vi "Scan_ctrl.vi"(0 "Scan Set up":T4={"Scan Type"=0, "Collection Information File Path"=path "", "Chemical"="Water", "Comments"="", "Collection Time / s"=60, "Number Acquires"=3, "How long to acquire"=75000000} {"Scan Type" items=["Normal Collection - 1 Colour", "Normal Collection - 2 Colour", "Delay Scan - 2 colour", "Accurate Delay Scan - 2 Colour", "Settings file"]}, 1 "Remote?":bool, 2 "appended path":path, 3 "Value":T5[](array[typedef]), 4 "Delay Cluster":T3={"System no."=0, "Identification"="", "Device ID out"=0, "Postion / mm"=[], "SN out"="", "Movement Range"=[], "Conn. Axes"=[], "Target Position / mm"=50.0, "Velocity / mm s^-1"=0.015, "Set-up"=FALSE, "Moving"=FALSE, "Step Size / mm "=0.15, "Stage Number"=0, "Polling Time /ms"=0, "Delay Scan?"=FALSE, "Accurate Scan"=FALSE, "CmdMovDelay"=FALSE, "CmdStopDelay"=FALSE, "Delay List"=[["Number", "Target / mm", "Relative Integration Time"]], "Scan Start /mm"=50.0, "Scan End / mm"=80.0, "Scan Velocity / mm s^-1"=0.15, "Delay Scan Time / s"=30.0}, 5 "error in (no error)":errorcluster, 6 "Remotepath":path) -> (7 "XML String Out":string, 8 "error out":errorcluster)   [LabVIEW 2018]
uses:
  Type defs/FileAcq_v1_Ctrl.ctl
  Type defs/Scan_ctrl.ctl
  Type defs/PI_delay_settings_alt.ctl
  Type defs/XML_info_TRPES.ctl
panel:
  in  "AcquistionInfo":T1
  in  "XMLcluster-TRPES":T2
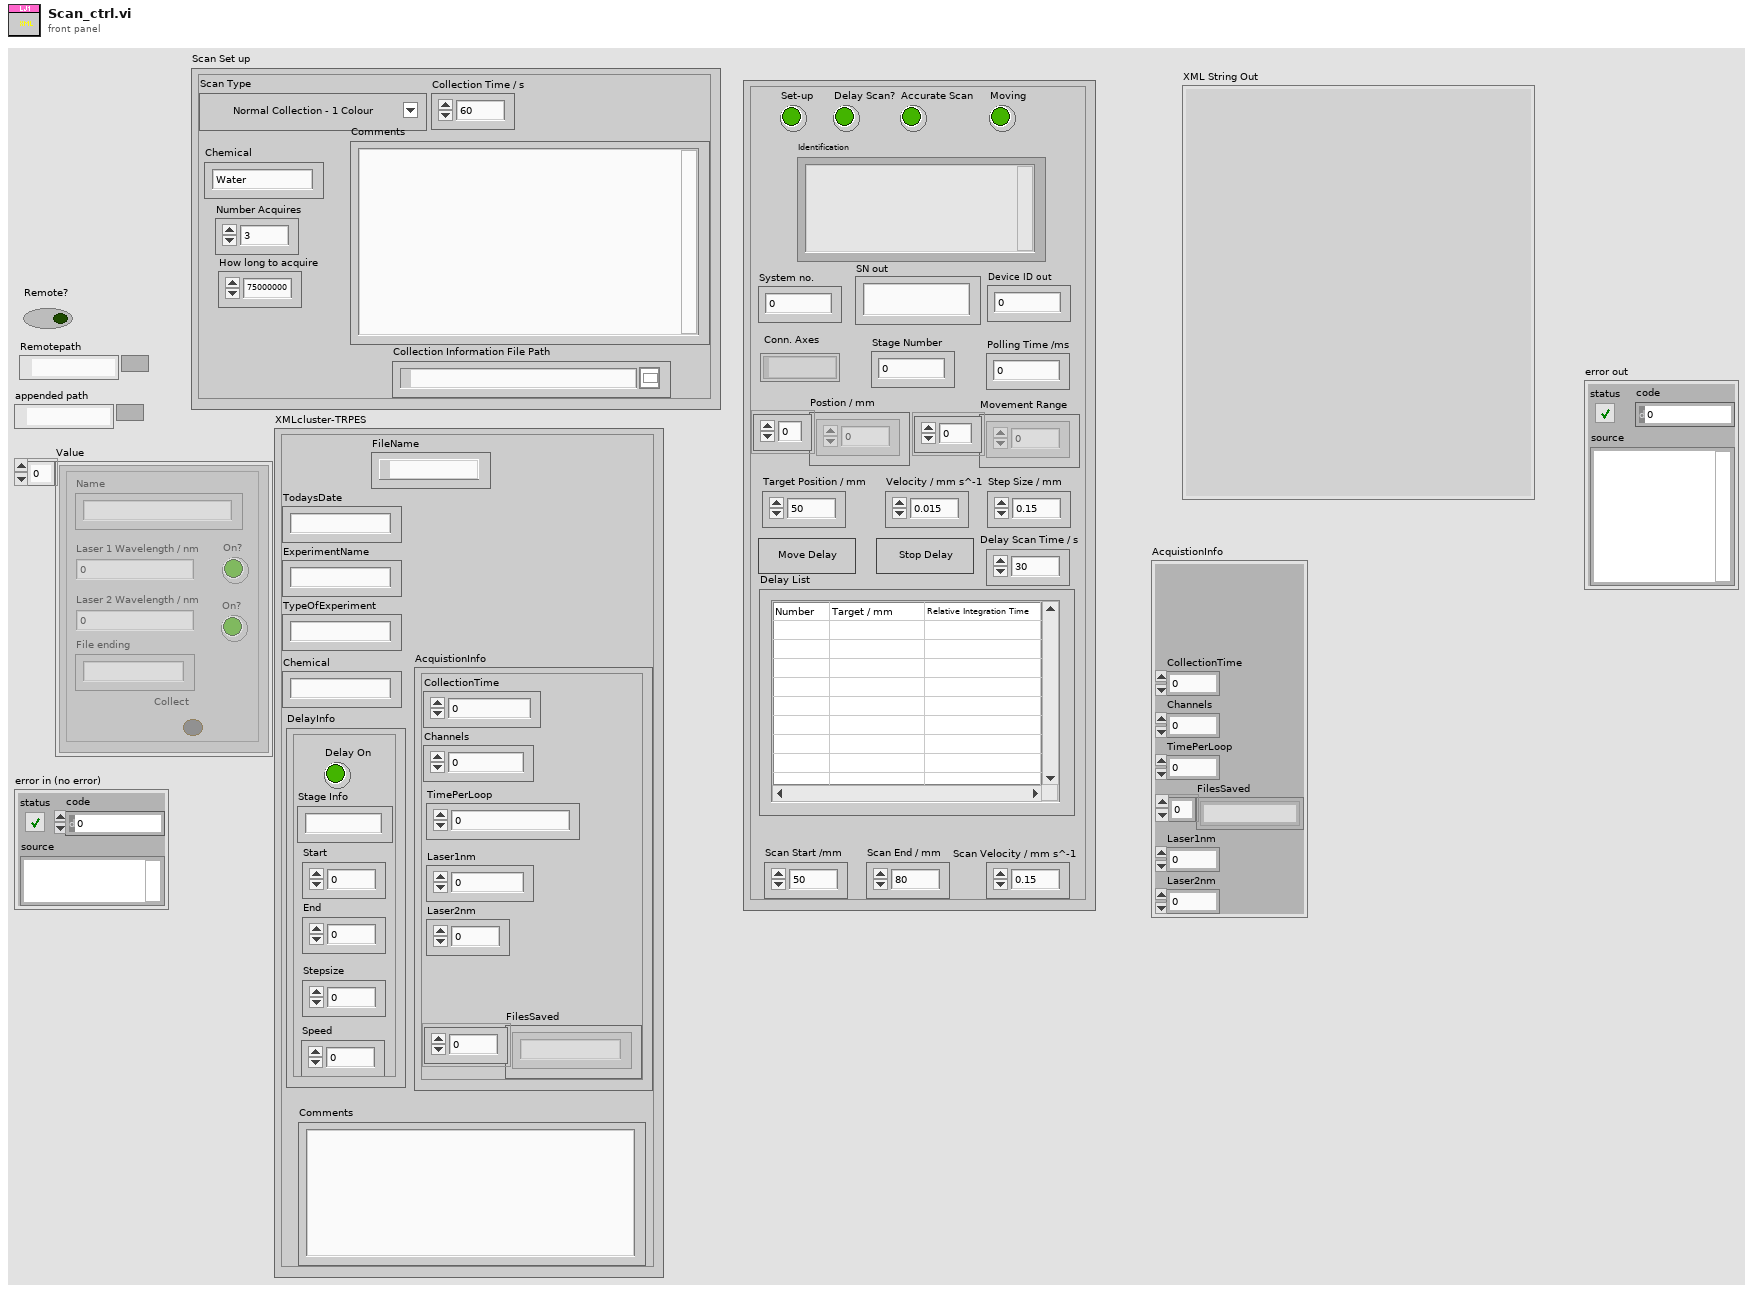
[diagram p1: front panel]
types:
  T1 = cluster{"CollectionTime":dbl, "Channels":dbl, "TimePerLoop":dbl, "FilesSaved":string[], "Laser1nm":dbl, "Laser2nm":dbl}
  T2 = typedef "XML_info_TRPES.ctl" = cluster{"FileName":path, "TodaysDate":string, "ExperimentName":string, "TypeOfExperiment":string, "AcquistionInfo":cluster{"CollectionTime":dbl, "Channels":dbl, "TimePerLoop":dbl, "FilesSaved":string[], "Laser1nm":dbl, "Laser2nm":dbl}, "Chemical":string, "DelayInfo":cluster{"Start":dbl, "End":dbl, "Stepsize":dbl, "Speed":dbl, "Stage Info":string, "Delay On":bool}, "Comments":string}
  T3 = typedef "PI_delay_settings_alt.ctl" = cluster{"System no.":i32, "Identification":string, "Device ID out":i32, "Postion / mm":dbl[], "SN out":string, "Movement Range":dbl[], "Conn. Axes":string[], "Target Position / mm":dbl, "Velocity / mm s^-1":dbl, "Set-up":bool, "Moving":bool, "Step Size / mm ":dbl, "Stage Number":i32, "Polling Time /ms":i32, "Delay Scan?":bool, "Accurate Scan":bool, "CmdMovDelay":bool, "CmdStopDelay":bool, "Delay List":string[][], "Scan Start /mm":dbl, "Scan End / mm":dbl, "Scan Velocity / mm s^-1":dbl, "Delay Scan Time / s":dbl}
  T4 = typedef "Scan_ctrl.ctl" = cluster{"Scan Type":u16, "Collection Information File Path":path, "Chemical":string, "Comments":string, "Collection Time / s":i32, "Number Acquires":i32, "How long to acquire":i32}
  T5 = typedef "FileAcq_v1_Ctrl.ctl" = cluster{"Type":string, "LaserWave1":dbl, "Shutter1":bool, "LaserWave2":dbl, "Shutter2":bool, "FileEnd":string, "Collect":bool}
  T6 = cluster{"Start":dbl, "End":dbl, "Stepsize":dbl, "Speed":dbl, "Stage Info":string, "Delay On":bool}
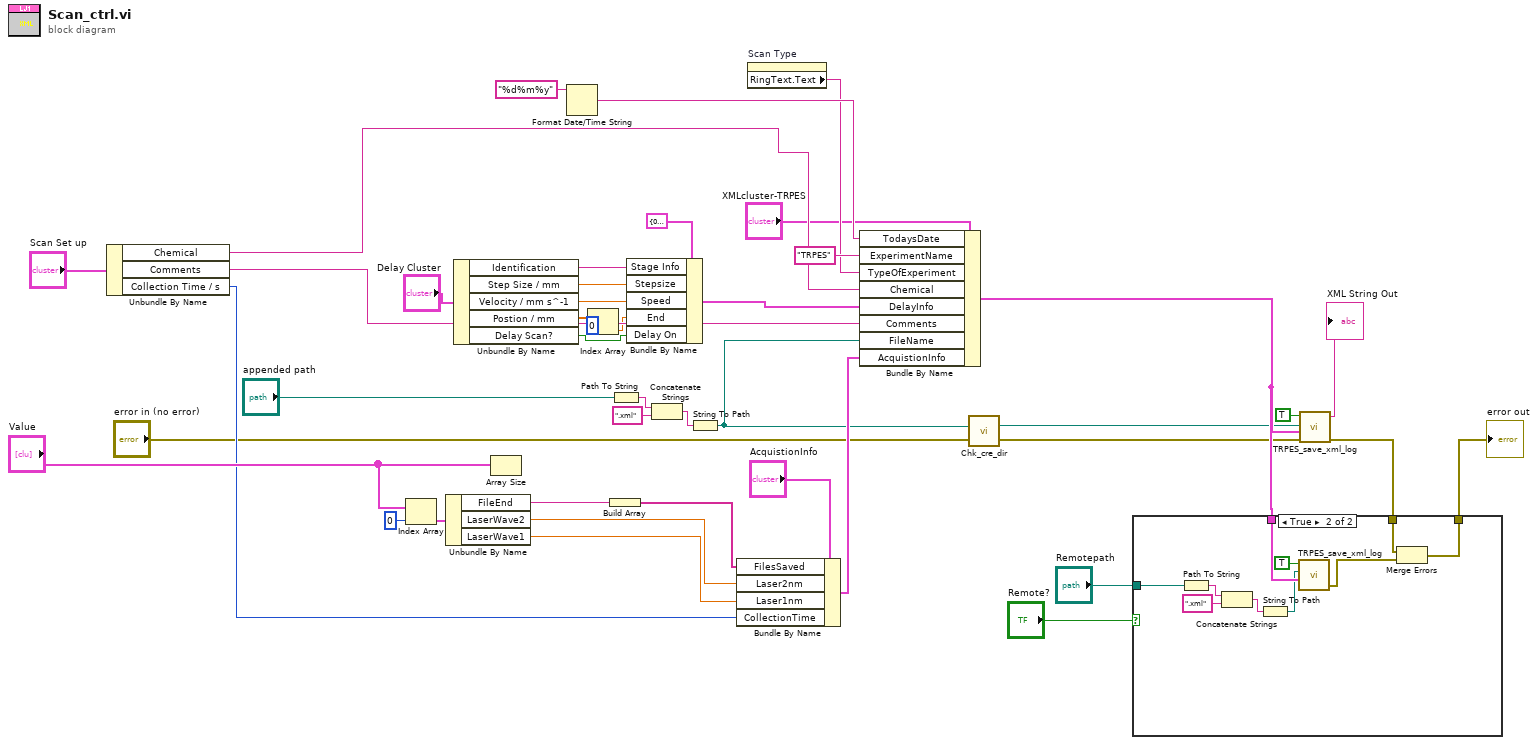
[diagram p0: block diagram]
diagram:
  n1 = Unbundle By Name("Scan Set up") -> ("Chemical"=w19:string, "Comments"=w18:string, "Collection Time / s"=w16:i32)
  n2 = Index Array(array="Value", index=0) -> (element=w30:T5)
  n3 = Unbundle By Name(w30) -> ("FileEnd"=w42:string, "LaserWave2"=w40:dbl, "LaserWave1"=w39:dbl)
  n4 = Unbundle By Name("Delay Cluster") -> ("Identification"=w32:string, "Step Size / mm"=w33:dbl, "Velocity / mm s^-1"=w34:dbl, "Postion / mm"=w15:dbl[], "Delay Scan?"=w10:bool)
  n5 = Array Size(array="Value") -> ()  [unwired: 1 out]
  n6 = Format Date/Time String(time format string (%c)="%d%m%y") -> (date/time string=w37:string)  [unwired: 2 in]
  n7 = Index Array(array=w15, index=0) -> (element=w14:dbl)
  n8 = Build Array(w42) -> (w43:string[])
  n9 = Path To String(path="appended path") -> (string=w23:string)
  n10 = Bundle By Name(cluster=T6 {"Start"=0.0, "End"=0.0, "Stepsize"=0.0, "Speed"=0.0, "Stage Info"="", "Delay On"=FALSE} ("DelayInfo"), "Stage Info"=w32, "Stepsize"=w33, "Speed"=w34, "End"=w14, "Delay On"=w10) -> (w35:T6)
  n11 = Concatenate Strings(w23, ".xml" ("string")) -> (w25:string)
  n12 = String To Path(string=w25) -> (path=w2:path)
  n13 = Bundle By Name(cluster="AcquistionInfo", "FilesSaved"=w43, "Laser2nm"=w40, "Laser1nm"=w39, "CollectionTime"=w16) -> (w11:T1)
  n14 = property on="Scan Type" class="Ring (strict)"() -> ("RingText.Text"=w20:string)  [unwired: 2 in, 2 out]
  n15 = Bundle By Name(cluster="XMLcluster-TRPES", "TodaysDate"=w37, "ExperimentName"="TRPES", "TypeOfExperiment"=w20, "Chemical"=w19, "DelayInfo"=w35, "Comments"=w18, "FileName"=w2, "AcquistionInfo"=w11) -> (w8:T2)
  n16 = call "Chk_cre_dir.vi"("error in (no error)"="error in (no error)", "Path"=w2) -> ("error out"=w3:errorcluster, "dup path"=w1:path)
  n17 = call "TRPES_save_xml_log.vi"("Error In"=w3, "XMLcluster-Jet"=w8, "XML File Path"=w1, "Write XML"=TRUE) -> ("Error Out"=w7:errorcluster, "XML String Out"=→"XML String Out":string)  [unwired: 1 in]
  n18 = case shown="True" "Remote?" {
    tunnel: w8 -> [_ w54]
    tunnel: w7 -> [w44 w51]
    tunnel: [w44 w50] -> w6
    tunnel: "Remotepath" -> [_ w45]
    frame False {
    }
    frame True {
      n19 = Path To String(path=w45) -> (string=w49:string)
      n20 = Concatenate Strings(w49, ".xml" ("string")) -> (w47:string)
      n21 = String To Path(string=w47) -> (path=w46:path)
      n22 = call "TRPES_save_xml_log.vi"("XMLcluster-Jet"=w54, "XML File Path"=w46, "Write XML"=TRUE) -> ("Error Out"=w52:errorcluster)  [unwired: 2 in, 1 out]
      n23 = Merge Errors(w51, w52) -> (w50:errorcluster)
    }
  }
  "error out" <- w6
